vi "Example Custom LVClass Serialization.vi"() -> ()   [LabVIEW 2019]
doc: "Example of injecting a custom serializer for conversion of LVClasses to JSON."
uses:
  Demo LVClass Serializer.lvclass
  C:/Users/Patrick/Documents/GitHub/Instrument-Framework/lvsrc/SMOs/JSON-RPC-2019/lv-venv/lv.lib/vi.lib/JDP Science/JSONtext/LVClass Serializer/JSONtext LVClass Serializer.lvclass
  <vilib>/ActorFramework/Message Enqueuer/Message Priority.ctl
  <vilib>/ActorFramework/Message Enqueuer/Message Enqueuer.lvclass
  <vilib>/ActorFramework/Message/Message.lvclass
  <vilib>/ActorFramework/Self-Addressed Msg/Self-Addressed Msg.lvclass/Self-Addressed Msg.ctl
  912a6c23-4bb1-4c3c-9308-e383c675d733.vi
  e1d0a090-eb0b-4084-98ba-e2f06df06374.vi
  vi.lib/JDP Science/JSONtext/Variant to JSON Text.vi
  vi.lib/JDP Science/JSONtext/JSON text to Variant.vi
  <vilib>/ActorFramework/Self-Addressed Msg/Self-Addressed Msg.lvclass
panel:
  out "Data out":T1
  out "x = y?":bool
  out "error out":errorcluster
  out "<JSON>":string
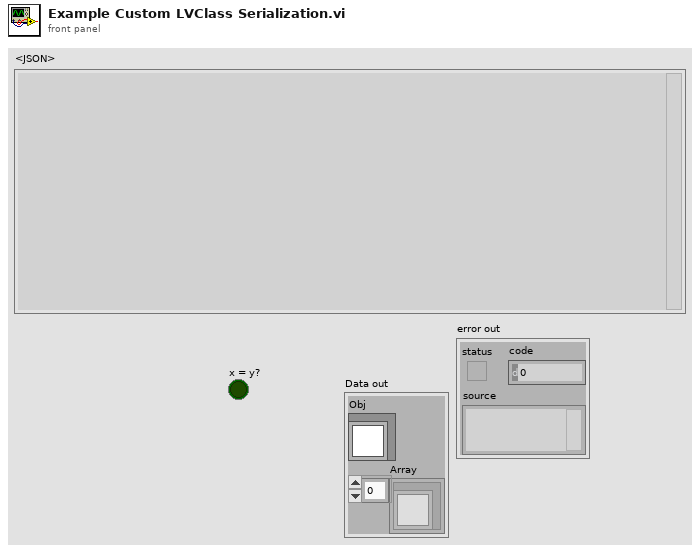
[diagram p1: front panel]
types:
  T1 = cluster{"Obj":refnum<class>, "Array":refnum<class>[]}
  T2 = typedef "Actor Framework.lvlib/Message Enqueuer.lvclass/Message Priority.ctl" = enum16{"Low", "Normal", "High"}
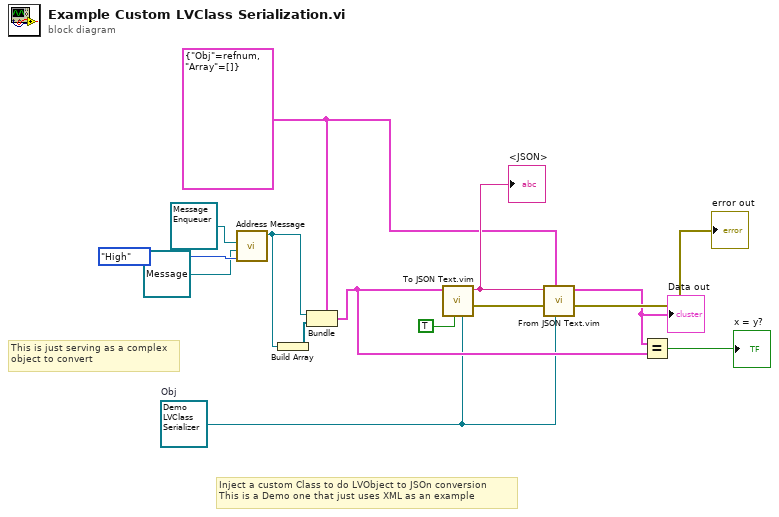
[diagram p0: block diagram]
diagram:
  w6 = T1 {"Obj"=refnum, "Array"=[]} ("output cluster")
  w5 = refnum<class "Demo LVClass Serializer.lvclass"> refnum  # Obj
  # "This is just serving as a complex\nobject to convert"
  # "Inject a custom Class to do LVObject to JSOn conversion\nThis is a Demo one that just uses XML as an example"
  n1 = call <vilib>:"Address Message.vi"("Message Priority (Normal)"=Message_Priority."High", "Message"=refnum<class "Message.lvclass"> refnum, "Destination"=refnum<class "Message Enqueuer.lvclass"> refnum) -> ("Self-Addressed Message"=w1:refnum<class "Self-Addressed Msg.lvclass">)  [unwired: 8 in]
  n2 = Build Array(w1) -> (w7:refnum<class "Self-Addressed Msg.lvclass">[])
  n3 = Bundle(cluster=w6, "Obj"=w1, "Array"=w7) -> (w9:T1)
  n4 = call "To JSON Text.vim"("LVClass Serializer"=w5, "Pretty Print?"=TRUE, "Anything"=w9) -> ("error out"=w12:errorcluster, "<JSON>"=w13:string)  [unwired: 7 in]
  "<JSON>" <- w13
  n5 = call "From JSON Text.vim"("LVClass Serializer"=w5, "Data Type and Default Value"=w6, "error in (no error)"=w12, "JSON"=w13) -> ("error out"=→"error out":errorcluster, "Data out"=w8:T1)  [unwired: 6 in]
  "Data out" <- w8
  n6 = Equal?(x=w8, y=w9) -> (x = y?=→"x = y?":bool)
